vi "PD_Filepath.vi"() -> ()   [LabVIEW 2009]
panel:
  in  "PD_Filepath":path
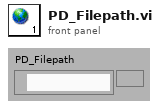
[diagram p1: front panel]
diagram:
